vi "Method 2.vi"(8 "error in (no error)":errorcluster, 10 "My Input":dbl, 11 "Test Actor 1 in":refnum<class "Test Async Actor.lvclass">) -> (0 "error out":errorcluster, 2 "My Output":dbl, 3 "Test Actor 1 out":refnum<class "Test Async Actor.lvclass">)   [LabVIEW 2023, in "Test Async Actor.lvlib" / "Test Async Actor.lvclass"]
doc: "My Method Description"
uses:
  Test Async Actor.lvclass
  Test Async Actor.lvclass/Test Async Actor.ctl
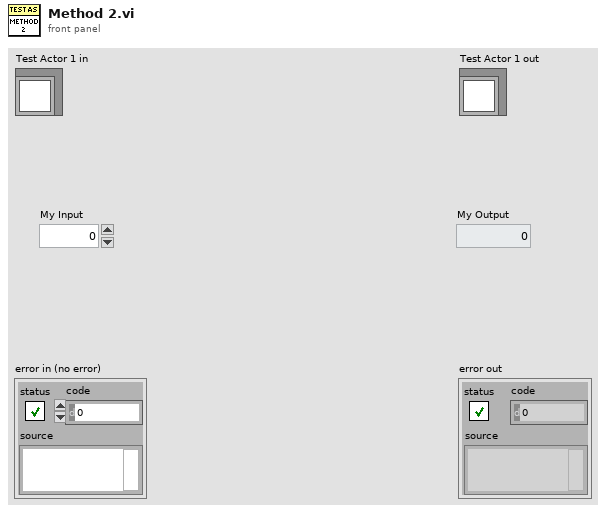
[diagram p1: front panel]
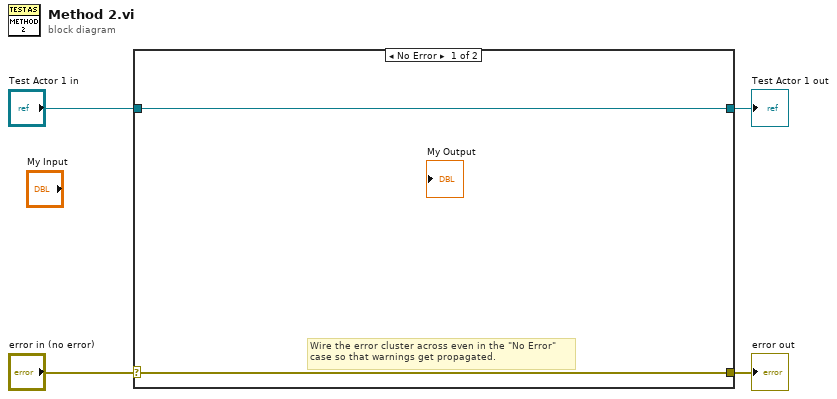
[diagram p0: block diagram]
diagram:
  n1 = case shown="No Error" "error in (no error)" {
    selector: "error in (no error)" -> [w5 w8]
    tunnel: [w5 w8] -> w3
    tunnel: [w6 w7] -> w1
    tunnel: "Test Actor 1 in" -> [w6 w7]
    frame No Error {
      # "Wire the error cluster across even in the \"No Error\"\ncase so that warnings get propagated."
    }
    frame Error {
    }
  }
  "error out" <- w3
  "Test Actor 1 out" <- w1
